vi "WinLSE_main.vi"(0 "N":dbl, 1 "Omega(t-1)":T1, 2 "y(t-1)":T1, 5 "x(t)":dbl, 7 "u(t)":dbl, 9 "dx/dt":dbl, 11 "error in (no error)":errorcluster, 13 "\\theta(t-1)":T1) -> (4 "\\theta(t)":T1, 6 "Omega(t)":T1, 8 "y(t)":T1, 15 "error out":errorcluster)   [LabVIEW 2021]
uses:
  <vilib>/Analysis/Matrix/Datatypes/RealMatrix.ctl
  <vilib>/Analysis/7linalg.llb/Eigenvalue and Vectors Output Option.ctl
  <vilib>/Analysis/_algsub.llb/Real PseudoInverse Matrix.vi
  <vilib>/Analysis/Matrix/Numeric/Multiply/Multiply - RM,RM.vi
  <vilib>/Analysis/7linalg.llb/Real Eigenvalues and Vectors.vi
  <vilib>/Analysis/Matrix/NI_Matrix.lvlib
  <vilib>/Analysis/NI_AALPro.lvlib
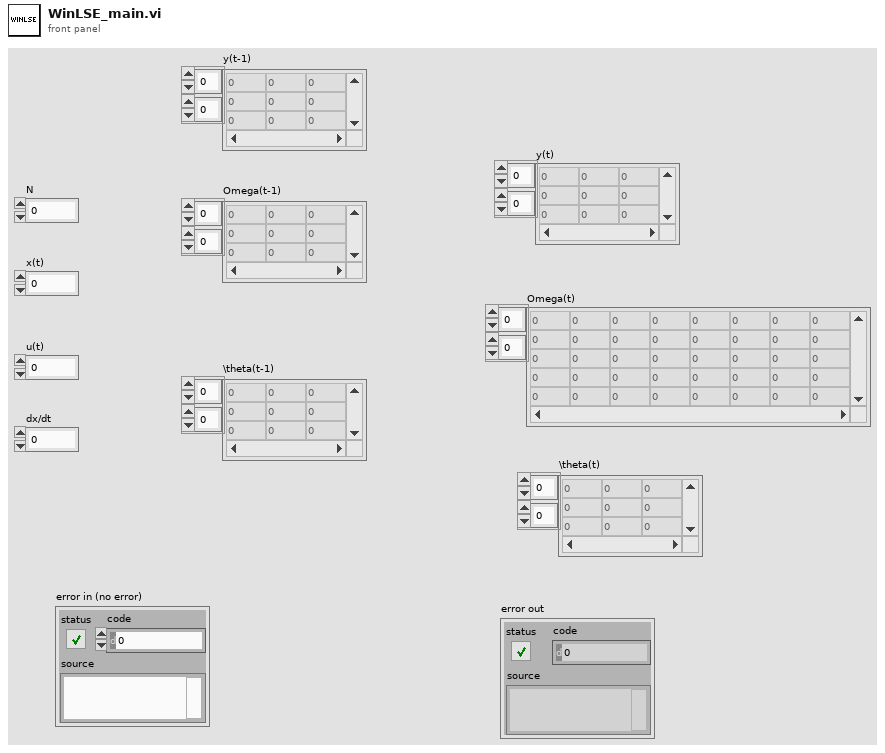
[diagram p1: front panel]
types:
  T1 = typedef "NI_Matrix.lvlib/RealMatrix.ctl" = dbl[][]
  T2 = typedef "NI_AALPro.lvlib/Eigenvalue and Vectors Output Option.ctl" = i32
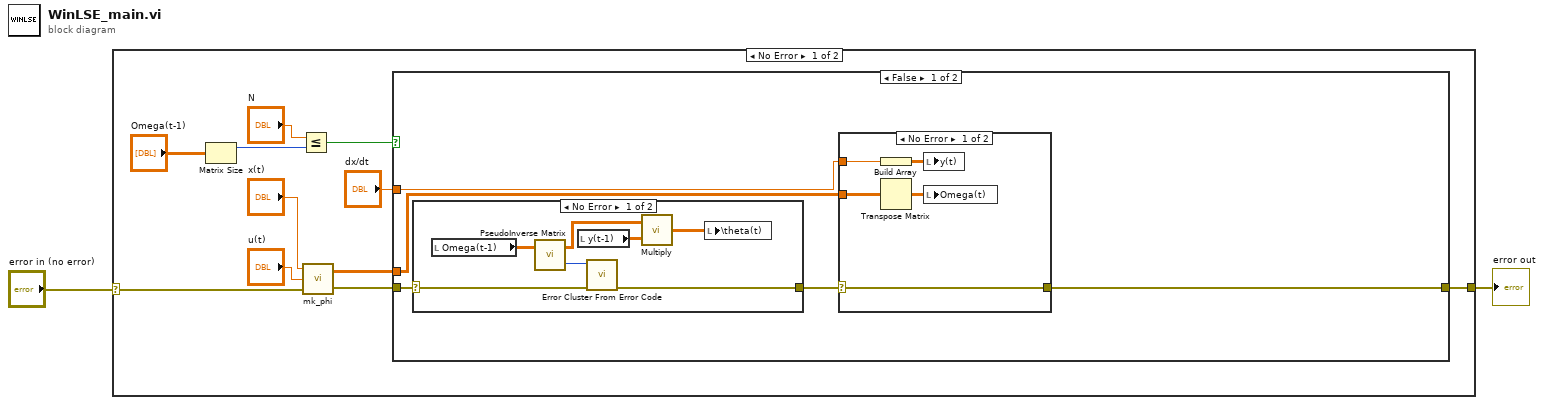
[diagram p0: block diagram]
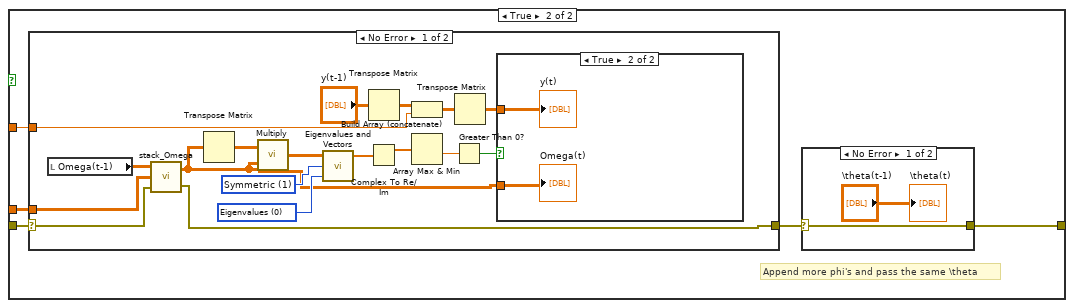
[diagram p4: hidden frame]
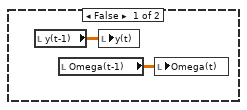
[diagram p6: hidden frame]
diagram:
  n1 = case shown="No Error" "error in (no error)" {
    selector: "error in (no error)" -> [w5 w64]
    tunnel: [w9 w64] -> w1
    frame No Error {
      n2 = Matrix Size(0:"Omega(t-1)") -> (1:w12:i32)  [unwired: 1 out]
      n3 = Less Or Equal?(x="N", y=w12) -> (x <= y?=w10:bool)
      n4 = call "mk_phi.vi"("error in (no error)"=w5, "u(t)"="u(t)", "x(t)"="x(t)") -> ("error out"=w4:errorcluster, "\\phi(t)"=w6:T1)
      n5 = case shown="False" w10 {
        tunnel: w4 -> [w18 w37]
        tunnel: [w14 w35] -> w9
        tunnel: w6 -> [w16 w34]
        tunnel: "dx/dt" -> [w15 w33]
        frame False {
          n6 = case shown="No Error" w18 {
            selector: w18 -> [w26 w32]
            tunnel: [w25 w32] -> w17
            frame No Error {
              n7 = local read "Omega(t-1)"() -> (w31:T1)
              n8 = call-poly <vilib>:"PseudoInverse Matrix.vi"("Input Matrix"=w31) -> ("error"=w27:i32, "PseudoInverse Matrix"=w30:T1)  [unwired: 1 in]
              n9 = local read "y(t-1)"() -> (w29:T1)
              n10 = call <vilib>:"Error Cluster From Error Code.vi"("error in (no error)"=w26, "error code (0)"=w27) -> ("error out"=w25:errorcluster)  [unwired: 7 in]
              n11 = call-poly <vilib>:"Multiply.vi"("Real Matrix B"=w29, "Real Matrix A"=w30) -> ("A * B"=w28:T1)
              n12 = local write "\\theta(t)"(w28) -> ()
            }
            frame Error {
            }
          }
          n13 = case shown="No Error" w17 {
            selector: w17 -> [w19 w24]
            tunnel: w16 -> [w22 _]
            tunnel: w15 -> [w20 _]
            tunnel: [w19 w24] -> w14
            frame No Error {
              n14 = Build Array(w20) -> (w21:T1)
              n15 = Transpose Matrix(1:w22) -> (0:w23:T1)
              n16 = local write "y(t)"(w21) -> ()
              n17 = local write "Omega(t)"(w23) -> ()
            }
            frame Error {
            }
          }
        }
        frame True {
          # "Append more phi's and pass the same \\theta"
          n18 = case shown="No Error" w37 {
            selector: w37 -> [w43 w63]
            tunnel: [w42 w63] -> w36
            tunnel: w34 -> [w44 _]
            tunnel: w33 -> [w41 _]
            frame No Error {
              w51 = T2 0 items=["Eigenvalues", "Eigenvalues & Vectors"] ("output option")
              w52 = 1 items=["General", "Symmetric"] ("matrix type")
              n19 = local read "Omega(t-1)"() -> (w58:T1)
              n20 = call "stack_Omega.vi"("error in (no error)"=w43, "\\phi(t)"=w44, "Omega"=w58) -> ("error out"=w42:errorcluster, "New Omega"=w45:T1)
              n21 = Transpose Matrix(1:w45) -> (0:w54:T1)
              n22 = call-poly <vilib>:"Multiply.vi"("Real Matrix B"=w45, "Real Matrix A"=w54) -> ("A * B"=w53:T1)
              n23 = call-poly <vilib>:"Eigenvalues and Vectors.vi"("output option"=w51, "matrix type"=w52, "Input Matrix"=w53) -> ("Eigenvalues"=w50:cdb[])  [unwired: 2 out]
              n24 = Transpose Matrix(1:"y(t-1)") -> (0:w55:T1)
              n25 = Complex To Re/Im(x + iy=w50) -> (x=w49:dbl[])  [unwired: 1 out]
              n26 = Build Array (concatenate)(w55, w41) -> (w57:T1)
              n27 = Array Max & Min(array=w49) -> (min value=w48:dbl)  [unwired: 3 out]
              n28 = Greater Than 0?(x=w48) -> (x > 0?=w47:bool)
              n29 = Transpose Matrix(1:w57) -> (0:w46:T1)
              n30 = case shown="True" w47 {
                tunnel: w46 -> [_ w62]
                tunnel: w45 -> [_ w61]
                frame False {
                  n31 = local read "y(t-1)"() -> (w59:T1)
                  n32 = local read "Omega(t-1)"() -> (w60:T1)
                  n33 = local write "y(t)"(w59) -> ()
                  n34 = local write "Omega(t)"(w60) -> ()
                }
                frame True {
                  "y(t)" <- w62
                  "Omega(t)" <- w61
                }
              }
            }
            frame Error {
            }
          }
          n35 = case shown="No Error" w36 {
            selector: w36 -> [w38 w40]
            tunnel: [w38 w40] -> w35
            frame No Error {
              "\\theta(t)" <- "\\theta(t-1)"
            }
            frame Error {
            }
          }
        }
      }
    }
    frame Error {
    }
  }
  "error out" <- w1
